vi "Grippers Example.vi"   [LabVIEW 2016]
doc: "Example VI: Opens and closes Baxter's grippers"
uses:
  ROS/Code/SubVIs/BaxterSide.ctl
  Devices/Baxter/BaxterVIs/LeftGripper.vi
panel:
  # "Hit run to close and open the gripper"
types:
  T1 = typedef "BaxterSide.ctl" = enum16{"left", "right"}
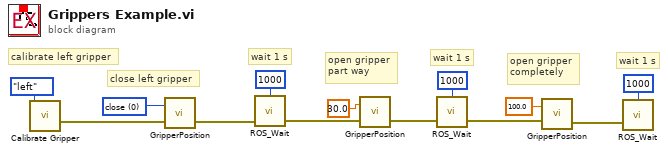
[diagram p0: block diagram]
diagram:
  w12 = u16 0 items=["close"=0, "open"=100] ("left gripper")
  # "wait 1 s"
  # "wait 1 s"
  # "wait 1 s"
  # "open gripper\ncompletely"
  # "open gripper\npart way"
  # "close left gripper"
  # "calibrate left gripper"
  n1 = call "Calibrate Gripper.vi"("Side"=BaxterSide."left") -> ("error out"=w11:errorcluster)  [unwired: 3 in]
  n2 = call-poly "GripperPosition.vi"("error in"=w11, "Desired Position"=w12) -> ("error out"=w8:errorcluster)  [unwired: 2 in]
  n3 = call "ROS_Wait.vi"("error in"=w8, "milliseconds to wait"=u32 1000) -> ("error out"=w7:errorcluster)  [unwired: 1 in, 1 out]
  n4 = call-poly "GripperPosition.vi"("error in"=w7, "Desired Position"=sgl 30.0) -> ("error out"=w4:errorcluster)  [unwired: 2 in]
  n5 = call "ROS_Wait.vi"("error in"=w4, "milliseconds to wait"=u32 1000) -> ("error out"=w3:errorcluster)  [unwired: 1 in, 1 out]
  n6 = call-poly "GripperPosition.vi"("error in"=w3, "Desired Position"=sgl 100.0) -> ("error out"=w1:errorcluster)  [unwired: 2 in]
  n7 = call "ROS_Wait.vi"("error in"=w1, "milliseconds to wait"=u32 1000) -> ()  [unwired: 1 in, 2 out]
